vi "Error Example_1.vi"() -> ()   [LabVIEW 2018]
doc: "This VI is an example and snippet showing error coding, with included call chain (reversed to show Top of Hierarchy first) and an ENUM that was not supported, encoded as a string.\n\n2010_10 Michael Ashe\nmichael.ashe@imaginatics.net\nImaginatics"
panel:
  in  "Some Enum":enum16{"First", "Second", "Third"}(ring)
  out "error out":errorcluster
  in  "error in (no error)":errorcluster
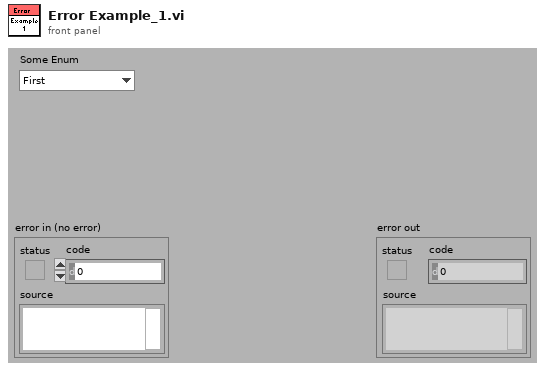
[diagram p1: front panel]
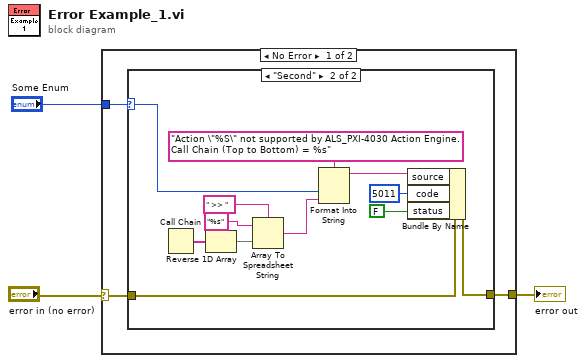
[diagram p0: block diagram]
diagram:
  n1 = case shown="No Error" "error in (no error)" {
    selector: "error in (no error)" -> [w6 _]
    tunnel: [w5 _] -> w2
    tunnel: "Some Enum" -> [w4 _]
    frame No Error {
      n2 = case shown="\"Second\"" w4 {
        selector: w4 -> [_ w7]
        tunnel: w6 -> [_ w9]
        tunnel: [_ w8] -> w5
        frame "First", Default {
        }
        frame "Second" {
          n3 = Call Chain() -> (call chain=w16:string[])
          n4 = Reverse 1D Array(array=w16) -> (reversed array=w10:string[])
          n5 = Array To Spreadsheet String(delimiter (Tab)=" >> ", array=w10, 3:"%s" ("format string")) -> (spreadsheet string=w14:string)
          n6 = Format Into String(format string="Action \"%S\" not supported by ALS_PXI-4030 Action Engine. Call Chain (Top to Bottom) = %s", w7, w14) -> (resulting string=w17:string)  [unwired: 2 in, 1 out]
          n7 = Bundle By Name(cluster=w9, "source"=w17, "code"=5011, "status"=FALSE) -> (w8:errorcluster)
        }
      }
    }
    frame Error {
    }
  }
  "error out" <- w2
